vi "Find Missing Elements in Array (String).vi"(10 "Full Array":T1[](array[typedef]), 11 "Partial Array":T1[](array[typedef])) -> (3 "Missing Elements":T1[](array[typedef]))   [LabVIEW 2018]
uses:
  <vilib>/ORNL/CSEISMIC DDS/CSEISMIC DDS Base/Data Types/Controls/DeviceID.ctl
  <vilib>/ORNL/CSEISMIC DDS/CSEISMIC DDS Base/CSEISMIC DDS.lvclass
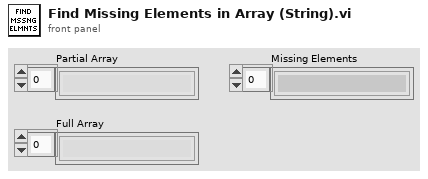
[diagram p1: front panel]
types:
  T1 = typedef "CSEISMIC DDS.lvlib/CSEISMIC DDS.lvclass/DeviceID.ctl" = string
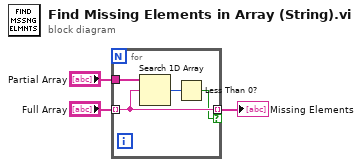
[diagram p0: block diagram]
diagram:
  n1 = for {
    tunnel: "Full Array" -> [w5] mode=indexing
    tunnel: "Partial Array" -> [w7]
    tunnel: [w5] -> w3 mode=indexing if=w4
    n2 = Search 1D Array(1D array=w7, element=w5) -> (index of element=w6:i32)  [unwired: 1 in]
    n3 = Less Than 0?(x=w6) -> (x < 0?=w4:bool)
  }
  "Missing Elements" <- w3
